vi "CSM - Replace Substitution Marks in Messages.vi"(5 "States With Replace Token":string, 7 "<param>":string, 9 "<target>":string, 12 "<1>":string, 13 "<2>":string) -> (6 "States":string)   [LabVIEW 2017, in "Communicable State Machine.lvlib"]
doc: "This VI is obsolete. Please use `CSM - Replace Marks in Messages.vi`\n\n### CSM - Replace Marks in Messages.vi\nFacilitates editing multiple CSM message strings by providing a batch replacement function for marks. There are four marks that can be replaced:\n- `<param>` mark: Usually represents the same argument.\n- `<target>` mark: Usually represents the same target.\n- `<1>` mark: Represents custom mark 1.\n- `<2>` mark: Represents custom mark 2.\n\n<b>Example</b>: The terminal `<target>` is connected to the string `DAQDevice`. The <b>States with Replace Token</b> string is:\n\n text\n Initialize -@ <target>\n Configure -@ <target>\n Read -@ <target>\n Close -@ <target>\n\nThe <b>States</b> output is:\n\n text\n Initialize -@ DAQDevice\n Configure -@ DAQDevice\n Read -@ DAQDevice\n Close -@ DAQDevice\n\n> - Ref: Message Building API\n\n-- <b>Controls</b> --\n- <b>States with Replace Token</b>: CSM state string with replacement marks.\n- <b><param></b>: `<param>` mark, which usually represents the same argument.\n- <b><target></b>: `<target>` mark, which usually represents the same target.\n- <b><1></b>: Custom mark 1.\n- <b><2></b>: Custom mark 2.\n\n-- <b>Indicators</b> --\n- <b>States</b>: State string after replacement."
uses:
  Communicable State Machine.lvlib
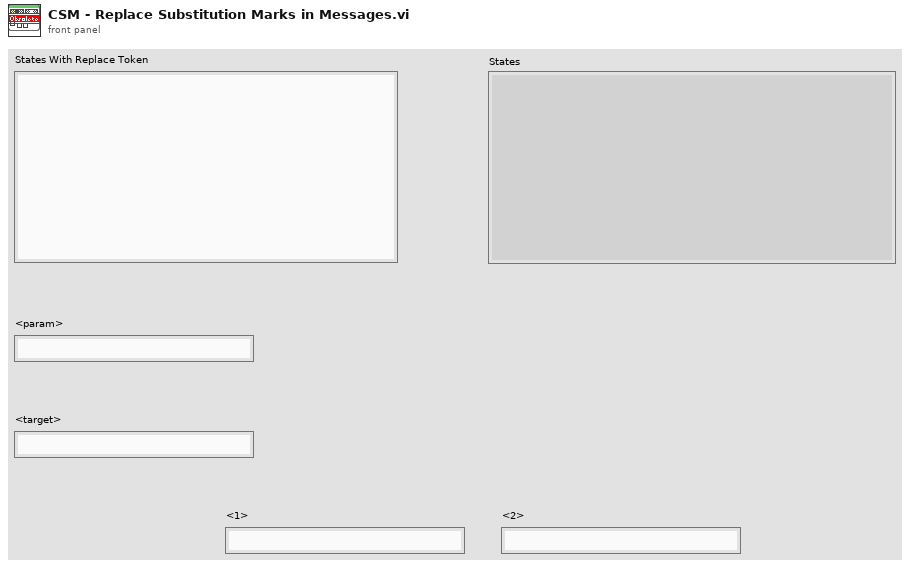
[diagram p1: front panel]
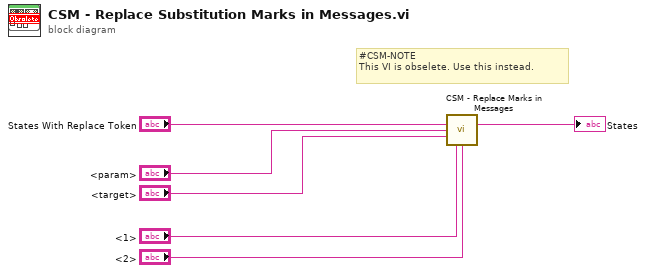
[diagram p0: block diagram]
diagram:
  # "#CSM-NOTE\nThis VI is obselete. Use this instead."
  n1 = call "CSM - Replace Marks in Messages.vi"("States With Replace Token"="States With Replace Token", "<param>"="<param>", "<target>"="<target>", "<1>"="<1>", "<2>"="<2>") -> ("States"=→"States":string)  [unwired: 10 in]
